vi "Write_Data.vi"(8 "error in (no error)":errorcluster caption="entrée d'erreur (pas d'erreur)", 10 "Data_To_Write":string, 11 "Class Relay_Board en entrée":refnum<class "Class Instrument Relay_Board.lvclass">) -> (0 "error out":errorcluster caption="sortie d'erreur", 3 "Class Relay_Board en Sortie":refnum<class "Class Instrument Relay_Board.lvclass">)   [LabVIEW 2020, in "Library Instrument & Equipement.lvlib" / "Library Instruments.lvlib" / "Class Instrument Relay_Board.lvclass"]
uses:
  Class Instrument Relay_Board.lvclass
  Commun VI/TypeDef/Commande Relay_Board/Data_Write_Relay_Board.ctl
  JSON API/JSON Value/Set from JSON string.vi
  JSON API/JSON Value/JSON Value.lvclass
  Class Instrument Relay_Board.lvclass/Class Instrument Relay_Board.ctl
  JSON API/Variant JSON/Variant JSON.lvlib
  JSON API/Get Polymorphic/JSON GetSet.lvlib
  Commun VI/Library Commun.lvlib
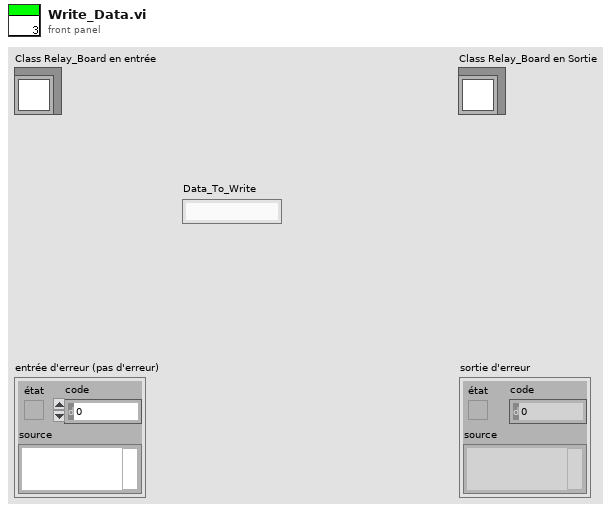
[diagram p1: front panel]
types:
  T1 = typedef "Library Commun.lvlib/Data_Write_Relay_Board.ctl" = enum16{"Enable Relays", "Disable Relays"}
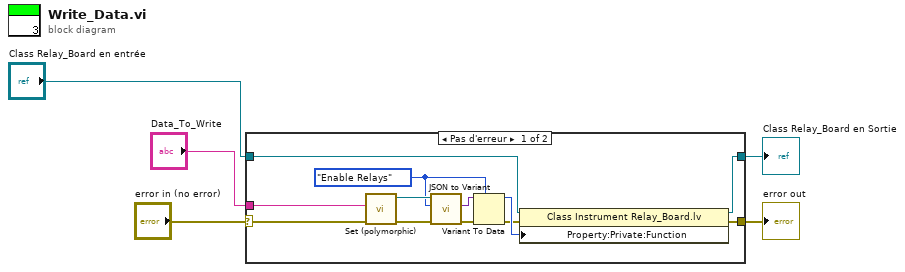
[diagram p0: block diagram]
diagram:
  n1 = case shown="Pas d'erreur" "error in (no error)" {
    selector: "error in (no error)" -> [w8 w19]
    tunnel: [w16 w19] -> w4
    tunnel: [w15 w18] -> w2
    tunnel: "Class Relay_Board en entrée" -> [w17 w18]
    tunnel: "Data_To_Write" -> [w10 _]
    frame No Error {
      w6 = Data_Write_Relay_Board."Enable Relays" ("Function")
      n2 = call-poly "Set (polymorphic).vi"("error in (no error)"=w8, "JSON stream"=w10) -> ("error out"=w13:errorcluster, "JSON Value out"=w11:refnum<class "JSON Value.lvclass">)  [unwired: 7 in, 1 out]
      n3 = call "JSON to Variant.vi"("error in (no error)"=w13, "Variant (Data Type)"=w6, "JSON Value"=w11) -> ("error out"=w12:errorcluster, "Variant out"=w14:variant)  [unwired: 7 in]
      n4 = Variant To Data(error in=w12, type=w6, Variant=w14) -> (data=w9:T1, error out=w7:errorcluster)
      n5 = property class="Class Instrument Relay_Board.lv"(reference=w17, error in=w7, "Property:Private:Function"=w9) -> (reference out=w15:refnum<class "Class Instrument Relay_Board.lvclass">, error out=w16:errorcluster)
    }
    frame Error {
    }
  }
  "error out" <- w4
  "Class Relay_Board en Sortie" <- w2
